vi "Puff_Analysis_AN.vi"(4 "Input Peak":dbl, 5 "Input Own Peak Value?":bool, 6 "Concentration":dbl[](array[numeric]), 7 "Time":dbl[](array[numeric])) -> (0 "Channel Values":string[](array[string]), 1 "Channel Names":string[](array[string]))   [LabVIEW 2015]
uses:
  <vilib>/Analysis/baseanly.llb/Mean (DBL).vi
  <vilib>/Analysis/NI_AALBase.lvlib
panel:
  out "Start":dbl
  out "End":dbl
  out "XY Graph":cluster{"Time":dbl[], "Concentration":dbl[]}[](graph)
  out "Decay Time":dbl
  out "50-50 Time":dbl
  out "Rise Time":dbl
  out "Fall Times":dbl[](array[numeric])
  out "Rise Times":dbl[](array[numeric])
  out "Peak Value":dbl
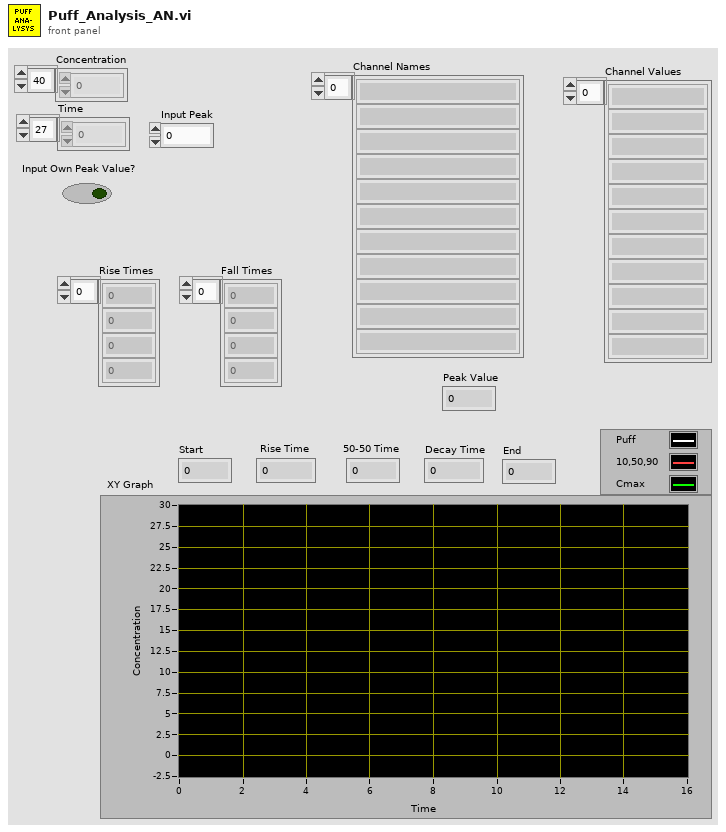
[diagram p1: front panel]
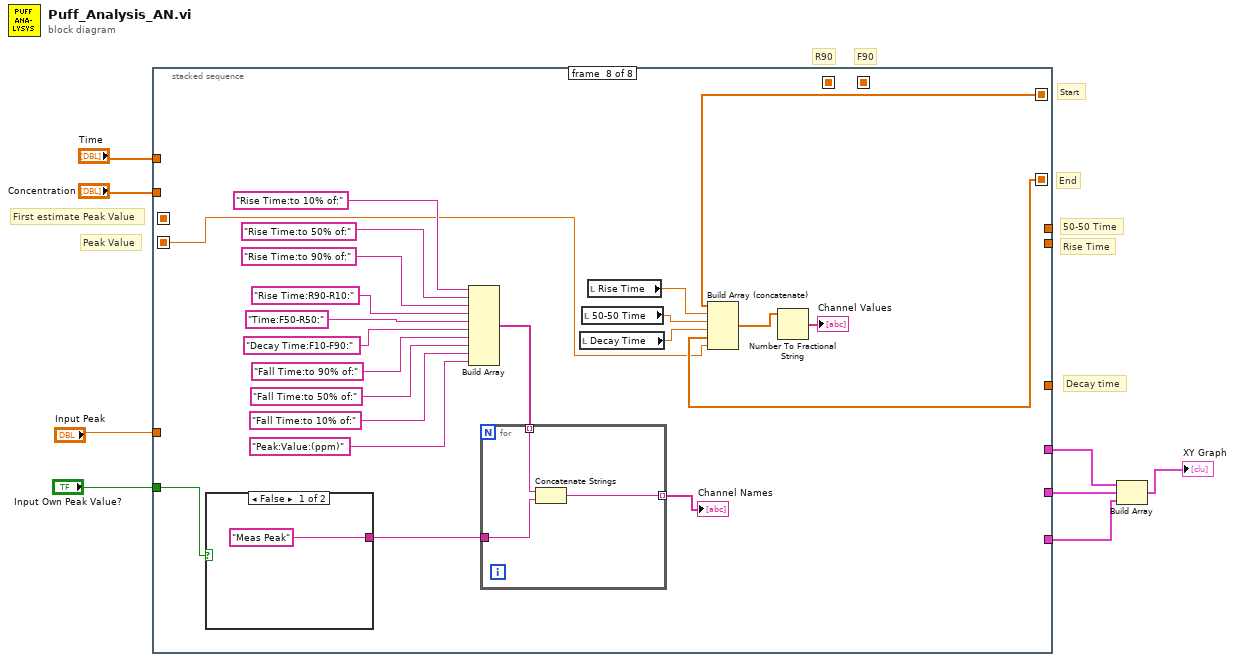
[diagram p0: block diagram]
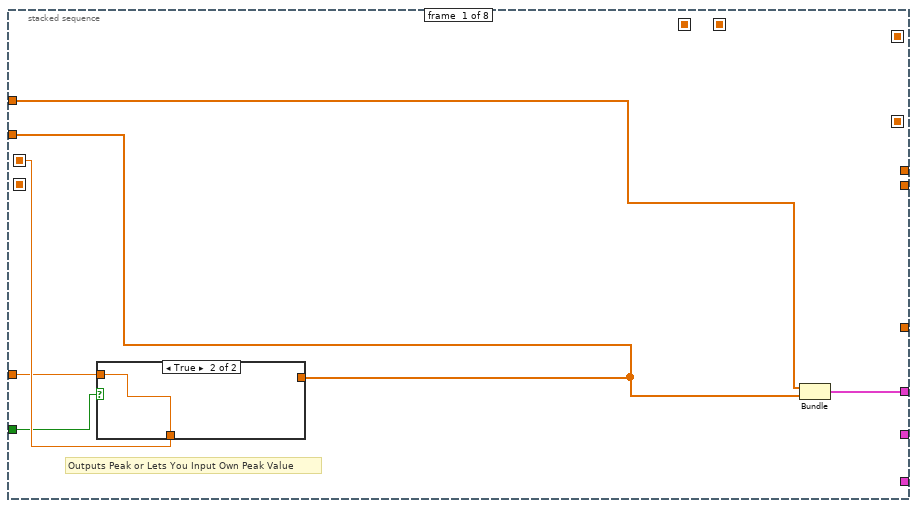
[diagram p2: hidden frame]
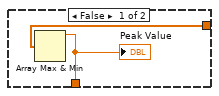
[diagram p3: hidden frame]
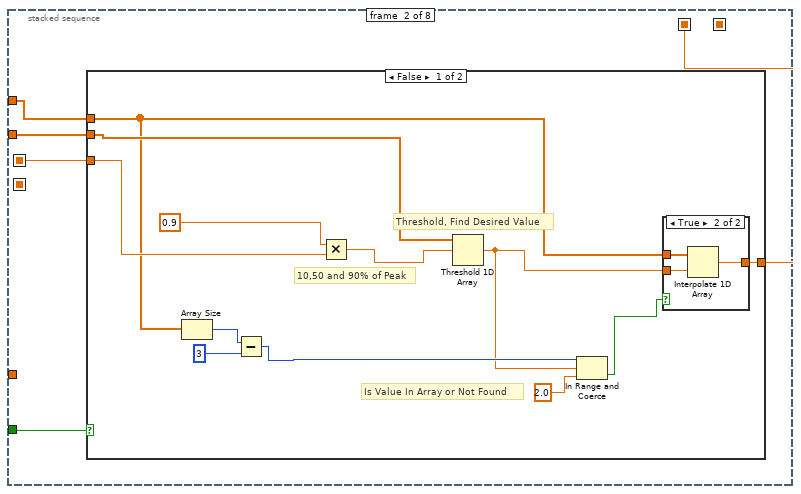
[diagram p4: hidden frame]
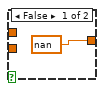
[diagram p5: hidden frame]
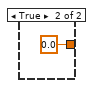
[diagram p6: hidden frame]
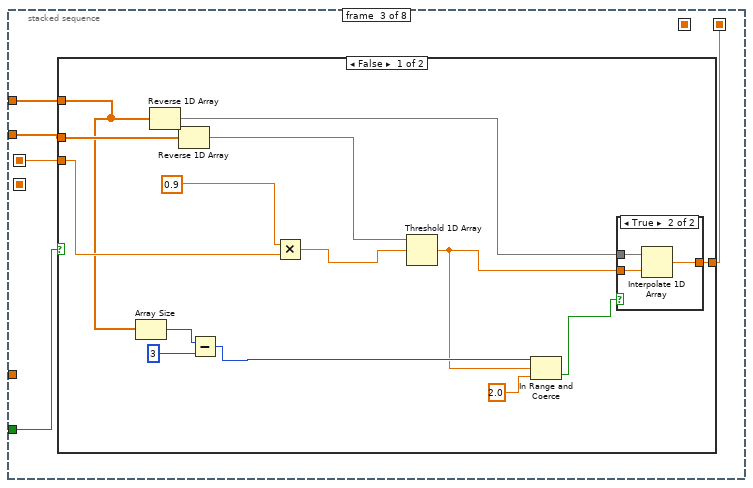
[diagram p7: hidden frame]
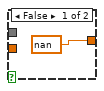
[diagram p8: hidden frame]
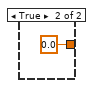
[diagram p9: hidden frame]
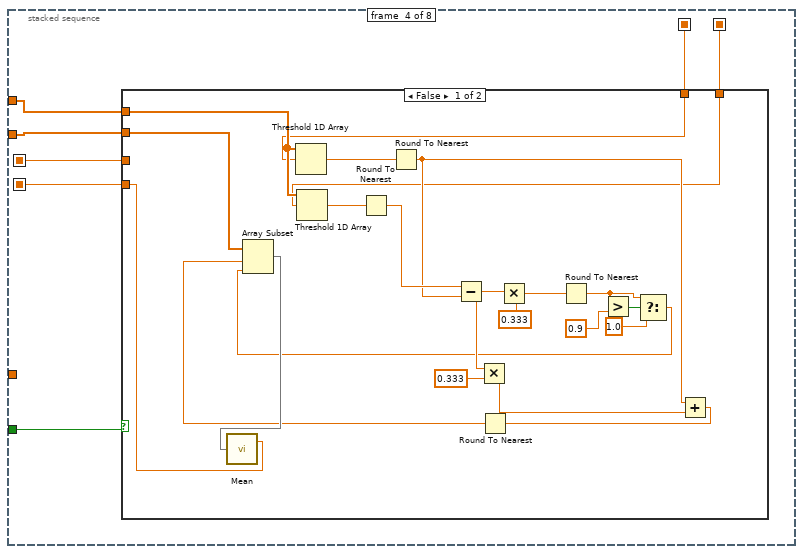
[diagram p10: hidden frame]
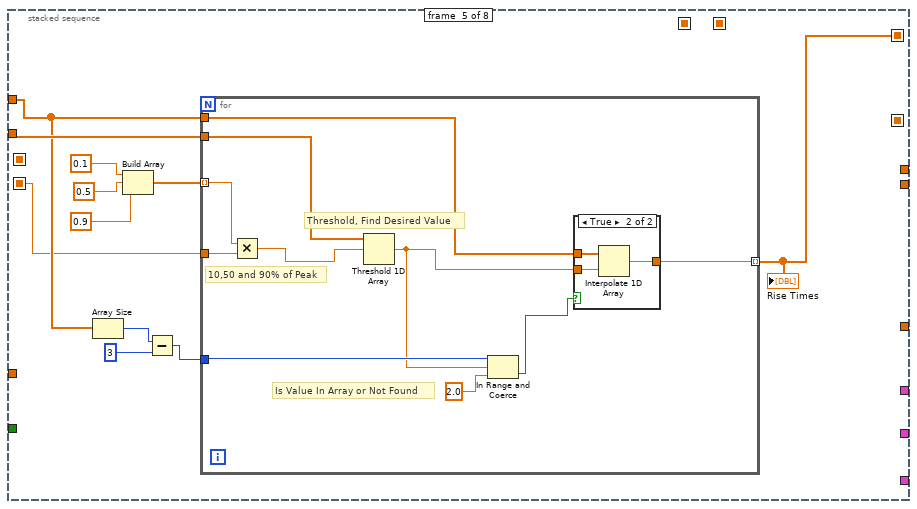
[diagram p12: hidden frame]
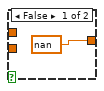
[diagram p13: hidden frame]
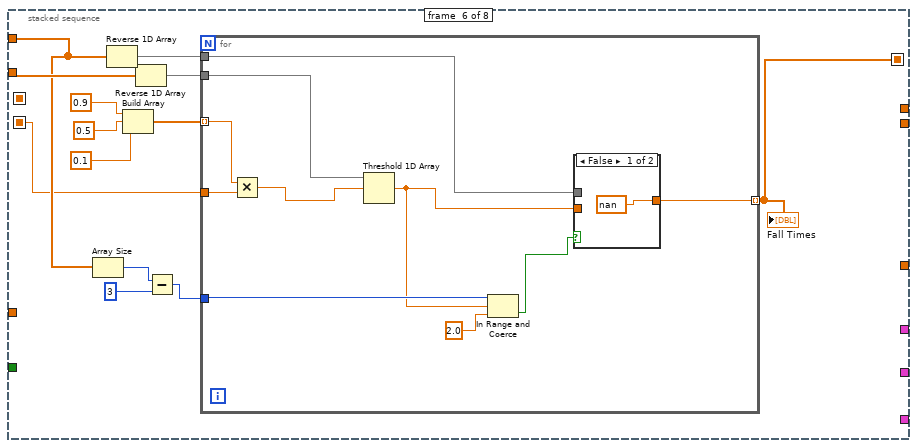
[diagram p14: hidden frame]
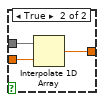
[diagram p15: hidden frame]
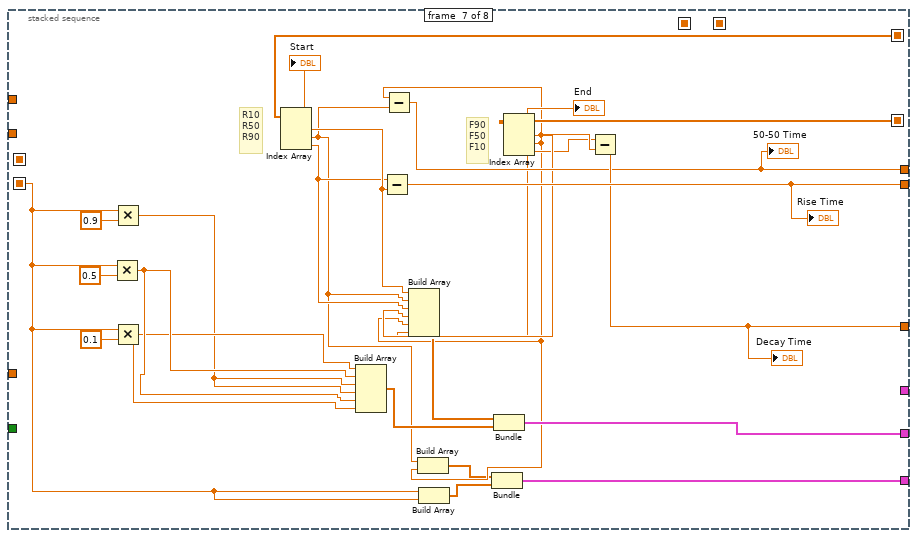
[diagram p16: hidden frame]
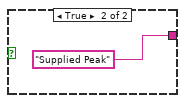
[diagram p17: hidden frame]
diagram:
  # "Peak Value"
  # "F90"
  # "R90"
  # "Decay time"
  # "Rise Time"
  # "50-50 Time"
  # "End"
  # "Start"
  # "First estimate Peak Value"
  n1 = stacked-sequence {
    seq-local: [w14 _ _ _ _ _ _ _] -> [_ w22 w44 w68 _ _ _ _]
    seq-local: [_ _ _ _ w100 _ _ _] -> [_ _ _ _ _ _ w169 w191]
    seq-local: [_ _ _ _ _ w122 _ _] -> [_ _ _ _ _ _ w168 w190]
    seq-local: [_ w19 _ _ _ _ _ _] -> [_ _ _ w65 _ _ _ _]
    seq-local: [_ _ w41 _ _ _ _ _] -> [_ _ _ w64 _ _ _ _]
    seq-local: [_ _ _ w69 _ _ _ _] -> [_ _ _ _ w94 w119 w146 w170]
    tunnel: [_ _ _ _ _ _ w165 _] -> _
    tunnel: [_ _ _ _ _ _ w167 _] -> _
    tunnel: [_ _ _ _ _ _ w166 _] -> _
    tunnel: [w13 _ _ _ _ _ _ _] -> w8
    tunnel: [_ _ _ _ _ _ w153 _] -> w6
    tunnel: [_ _ _ _ _ _ w147 _] -> w5
    tunnel: "Time" -> [w12 w20 w42 w66 w95 w120 _ _]
    tunnel: "Concentration" -> [w11 w21 w43 w67 w96 w121 _ _]
    tunnel: "Input Own Peak Value?" -> [w10 w18 w40 w70 _ _ _ w175]
    tunnel: "Input Peak" -> [w9 _ _ _ _ _ _ _]
    frame #0 {
      # "Outputs Peak or Lets You Input Own Peak Value"
      n2 = case shown="True" w10 {
        tunnel: [w16 w17] -> w14
        tunnel: w11 -> [w15 _]
        tunnel: w9 -> [_ w17]
        frame False {
          n3 = Array Max & Min(array=w15) -> (max value=w16:dbl)  [unwired: 3 out]
          "Peak Value" <- w16
        }
        frame True {
        }
      }
      n4 = Bundle("Time"=w12, "Concentration"=w11) -> (w13:cluster{"Time":dbl[], "Concentration":dbl[]})  [unwired: 1 in]
    }
    frame #1 {
      n5 = case shown="False" w18 {
        tunnel: w22 -> [w34 _]
        tunnel: w21 -> [w30 _]
        tunnel: w20 -> [w29 _]
        tunnel: [w28 0.0] -> w19
        frame False {
          # "10,50 and 90% of Peak"
          # "Is Value In Array or Not Found"
          # "Threshold, Find Desired Value"
          n6 = Array Size(array=w29) -> (size(s)=w32:i32)
          n7 = Subtract(x=w32, y=3) -> (x-y=w31:i32)
          n8 = Multiply(x=0.9 ("y"), y=w34) -> (x*y=w27:dbl)
          n9 = Threshold 1D Array(2:w27, 3:w30) -> (0:w24:dbl)  [unwired: 1 in]
          n10 = In Range and Coerce(upper limit=w31, x=w24, lower limit=2.0) -> (In Range?=w25:bool)  [unwired: 1 out]
          n11 = case shown="True" w25 {
            tunnel: w24 -> [_ w38]
            tunnel: [nan w37] -> w28
            tunnel: w29 -> [_ w36]
            frame False {
            }
            frame True {
              n12 = Interpolate 1D Array(1:w38, 2:w36) -> (0:w37:dbl)
            }
          }
        }
        frame True {
        }
      }
    }
    frame #2 {
      n13 = case shown="False" w40 {
        tunnel: w44 -> [w58 _]
        tunnel: w43 -> [w52 _]
        tunnel: w42 -> [w51 _]
        tunnel: [w45 0.0] -> w41
        frame False {
          n14 = Array Size(array=w51) -> (size(s)=w56:i32)
          n15 = Reverse 1D Array(array=w51) -> (reversed array=w54:dbl[])
          n16 = Reverse 1D Array(array=w52) -> (reversed array=w53:dbl[])
          n17 = Subtract(x=w56, y=3) -> (x-y=w55:i32)
          n18 = Multiply(x=0.9 ("y"), y=w58) -> (x*y=w50:dbl)
          n19 = Threshold 1D Array(2:w50, 3:w53) -> (0:w47:dbl)  [unwired: 1 in]
          n20 = In Range and Coerce(upper limit=w55, x=w47, lower limit=2.0) -> (In Range?=w48:bool)  [unwired: 1 out]
          n21 = case shown="True" w48 {
            tunnel: w47 -> [_ w62]
            tunnel: [nan w61] -> w45
            tunnel: w54 -> [_ w60]
            frame False {
            }
            frame True {
              n22 = Interpolate 1D Array(1:w62, 2:w60) -> (0:w61:dbl)
            }
          }
        }
        frame True {
        }
      }
    }
    frame #3 {
      n23 = case shown="False" w70 {
        tunnel: [w79 w93] -> w69
        tunnel: w68 -> [_ w93]
        tunnel: w67 -> [w92 _]
        tunnel: w66 -> [w90 _]
        tunnel: w65 -> [w78 _]
        tunnel: w64 -> [w77 _]
        frame False {
          n24 = Threshold 1D Array(2:w78, 3:w90) -> (0:w91:dbl)  [unwired: 1 in]
          n25 = Threshold 1D Array(2:w77, 3:w90) -> (0:w89:dbl)  [unwired: 1 in]
          n26 = Round To Nearest(number=w89) -> (nearest integer value=w88:dbl)
          n27 = Round To Nearest(number=w91) -> (nearest integer value=w82:dbl)
          n28 = Subtract(x=w88, y=w82) -> (x-y=w85:dbl)
          n29 = Multiply(x=w85, y=0.333) -> (x*y=w83:dbl)
          n30 = Multiply(x=w85, y=0.333) -> (x*y=w86:dbl)
          n31 = Round To Nearest(number=w86) -> (nearest integer value=w73:dbl)
          n32 = Greater?(x=w73, y=0.9) -> (0:w74:bool)
          n33 = Select(t=w73, s=w74, f=1.0) -> (s? t:f=w71:dbl)
          n34 = Add(x=w82, y=w83) -> (x+y=w81:dbl)
          n35 = Round To Nearest(number=w81) -> (nearest integer value=w76:dbl)
          n36 = Array Subset(array=w92, index=w76, length=w71) -> (w80:dbl[])
          n37 = call-poly <vilib>:"Mean.vi"("X"=w80) -> ("mean"=w79:dbl)  [unwired: 1 out]
        }
        frame True {
        }
      }
    }
    frame #4 {
      n38 = Array Size(array=w95) -> (size(s)=w98:i32)
      n39 = Build Array(0.1 ("y"), 0.5 ("y"), 0.9 ("y")) -> (w101:dbl[])
      n40 = Subtract(x=w98, y=3) -> (x-y=w97:i32)
      n41 = for {
        tunnel: w101 -> [w112] mode=indexing
        tunnel: w94 -> [w113]
        tunnel: w95 -> [w109]
        tunnel: w96 -> [w110]
        tunnel: [w111] -> w100 mode=indexing
        tunnel: w97 -> [w108]
        # "10,50 and 90% of Peak"
        # "Is Value In Array or Not Found"
        # "Threshold, Find Desired Value"
        n42 = Multiply(x=w112, y=w113) -> (x*y=w114:dbl)
        n43 = Threshold 1D Array(2:w114, 3:w110) -> (0:w105:dbl)  [unwired: 1 in]
        n44 = In Range and Coerce(upper limit=w108, x=w105, lower limit=2.0) -> (In Range?=w106:bool)  [unwired: 1 out]
        n45 = case shown="True" w106 {
          tunnel: w105 -> [_ w118]
          tunnel: [nan w117] -> w111
          tunnel: w109 -> [_ w116]
          frame False {
          }
          frame True {
            n46 = Interpolate 1D Array(1:w118, 2:w116) -> (0:w117:dbl)
          }
        }
      }
      "Rise Times" <- w100
    }
    frame #5 {
      n47 = Array Size(array=w120) -> (size(s)=w126:i32)
      n48 = Reverse 1D Array(array=w120) -> (reversed array=w124:dbl[])
      n49 = Build Array(0.9 ("y"), 0.5 ("y"), 0.1 ("y")) -> (w128:dbl[])
      n50 = Reverse 1D Array(array=w121) -> (reversed array=w123:dbl[])
      n51 = Subtract(x=w126, y=3) -> (x-y=w125:i32)
      n52 = for {
        tunnel: w128 -> [w139] mode=indexing
        tunnel: w119 -> [w140]
        tunnel: w124 -> [w136]
        tunnel: w123 -> [w137]
        tunnel: [w138] -> w122 mode=indexing
        tunnel: w125 -> [w135]
        n53 = Multiply(x=w139, y=w140) -> (x*y=w141:dbl)
        n54 = Threshold 1D Array(2:w141, 3:w137) -> (0:w132:dbl)  [unwired: 1 in]
        n55 = In Range and Coerce(upper limit=w135, x=w132, lower limit=2.0) -> (In Range?=w133:bool)  [unwired: 1 out]
        n56 = case shown="False" w133 {
          tunnel: w132 -> [_ w145]
          tunnel: [nan w144] -> w138
          tunnel: w136 -> [_ w143]
          frame False {
          }
          frame True {
            n57 = Interpolate 1D Array(1:w145, 2:w143) -> (0:w144:dbl)
          }
        }
      }
      "Fall Times" <- w122
    }
    frame #6 {
      # "R10\nR50\nR90"
      # "F90\nF50\nF10"
      n58 = Multiply(x=w146, y=0.5) -> (x*y=w161:dbl)
      n59 = Multiply(x=w146, y=0.9) -> (x*y=w150:dbl)
      n60 = Multiply(x=w146, y=0.1) -> (x*y=w160:dbl)
      n61 = Index Array(array=w169) -> (element #1=w159:dbl, element #2=w152:dbl, element #3=w158:dbl)  [unwired: 3 in]
      "Start" <- w159
      n62 = Build Array(w160, w161, w150, w150, w161, w160) -> (w154:dbl[])
      n63 = Subtract(x=w158, y=w159) -> (x-y=w167:dbl)
      "Rise Time" <- w167
      n64 = Build Array(w146, w146) -> (w149:dbl[])
      n65 = Index Array(array=w168) -> (element #1=w157:dbl, element #2=w151:dbl, element #3=w156:dbl)  [unwired: 3 in]
      "End" <- w157
      n66 = Subtract(x=w151, y=w152) -> (x-y=w165:dbl)
      "50-50 Time" <- w165
      n67 = Build Array(w159, w152, w158, w157, w151, w156) -> (w155:dbl[])
      n68 = Build Array(w152, w151) -> (w148:dbl[])
      n69 = Bundle(w148, w149) -> (w147:cluster{dbl[], dbl[]})  [unwired: 1 in]
      n70 = Bundle(w155, w154) -> (w153:cluster{dbl[], dbl[]})  [unwired: 1 in]
      n71 = Subtract(x=w156, y=w157) -> (x-y=w166:dbl)
      "Decay Time" <- w166
    }
    frame #7 {
      n72 = case shown="False" w175 {
        tunnel: ["Meas Peak" "Supplied Peak"] -> w174
        frame False {
        }
        frame True {
        }
      }
      n73 = Build Array("Rise Time:to 10% of:", "Rise Time:to 50% of:", "Rise Time:to 90% of:", "Rise Time:R90-R10:", "Time:F50-R50:", "Decay Time:F10-F90:", "Fall Time:to 90% of:", "Fall Time:to 50% of:", "Fall Time:to 10% of:", "Peak:Value:(ppm)") -> (w173:string[])
      n74 = for {
        tunnel: w174 -> [w196]
        tunnel: w173 -> [w195] mode=indexing
        tunnel: [w194] -> w172 mode=indexing
        n75 = Concatenate Strings(w195, w196) -> (w194:string)
      }
      "Channel Names" <- w172
      n76 = local read "Decay Time"() -> (w187:dbl)
      n77 = local read "50-50 Time"() -> (w188:dbl)
      n78 = local read "Rise Time"() -> (w189:dbl)
      n79 = Build Array (concatenate)(w191, w189, w188, w187, w190, w170) -> (w177:dbl[])
      n80 = Number To Fractional String(number=w177) -> (F-format string=→"Channel Values":string[])  [unwired: 3 in]
    }
  }
  n81 = Build Array(w8, w6, w5) -> (→"XY Graph":cluster{"Time":dbl[], "Concentration":dbl[]}[])
